vi "Get Storage Reference.vi"(8 "error in (no error)":errorcluster, 11 "Result in":refnum<class "Task.lvclass">) -> (0 "error out":errorcluster, 3 "notifier":refnum<notifier>)   [LabVIEW 2017, in "Futures.lvlib" / "Task.lvclass"]
uses:
  Task.lvclass
  Task Data.ctl
  Task State.ctl
  Task.lvclass/Task.ctl
  <vilib>/Utility/error.llb/Error Cluster From Error Code.vi
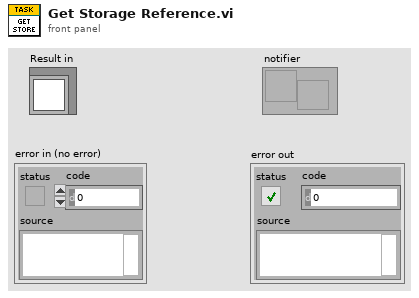
[diagram p1: front panel]
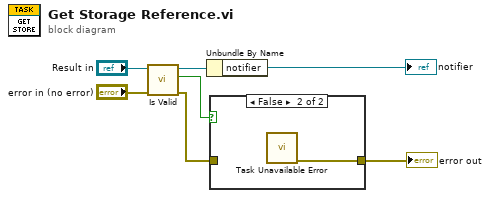
[diagram p0: block diagram]
diagram:
  n1 = call "Is Valid.vi"("error in (no error)"="error in (no error)", "Result in"="Result in") -> ("error out"=w2:errorcluster, "Valid"=w3:bool, "Result out"=w5:refnum<class "Task.lvclass">)  [unwired: 7 in]
  n2 = Unbundle By Name(w5) -> ("notifier"=→"notifier":refnum<notifier>)
  n3 = case shown="False" w3 {
    tunnel: w2 -> [w8 _]
    tunnel: [w8 w9] -> w1
    frame True {
    }
    frame False {
      n4 = call "Task Unavailable Error.vi"() -> ("error out"=w9:errorcluster)  [unwired: 11 in]
    }
  }
  "error out" <- w1
